vi "Step 8.vi"(8 "error in (no error)":errorcluster, 11 "HeatUp Data in":string[][](array[string])) -> (0 "error out":errorcluster, 1 "Min-Run Evap Temp (T3A)":dbl, 2 "EEV":u32, 3 "Evaporator Superheat (Deg F)":dbl format="%#.4g", 4 "Evaporator Superheat":T1(graph), 5 "Min-Run Evap Temp (T3A)":T1(graph), 7 "EEV":T1(graph))   [LabVIEW 2019]
uses:
  <vilib>/Utility/error.llb/DialogType.ctl
panel:
  out "error out 2":errorcluster
  in  "error in (no error) 2":errorcluster
  out "120 Array":dbl[][](array[numeric])
  out "transposed array":dbl[][](array[numeric])
  out "HeatUp Data in 2":string[][](array[string])
  # "Data with Stripped Header"
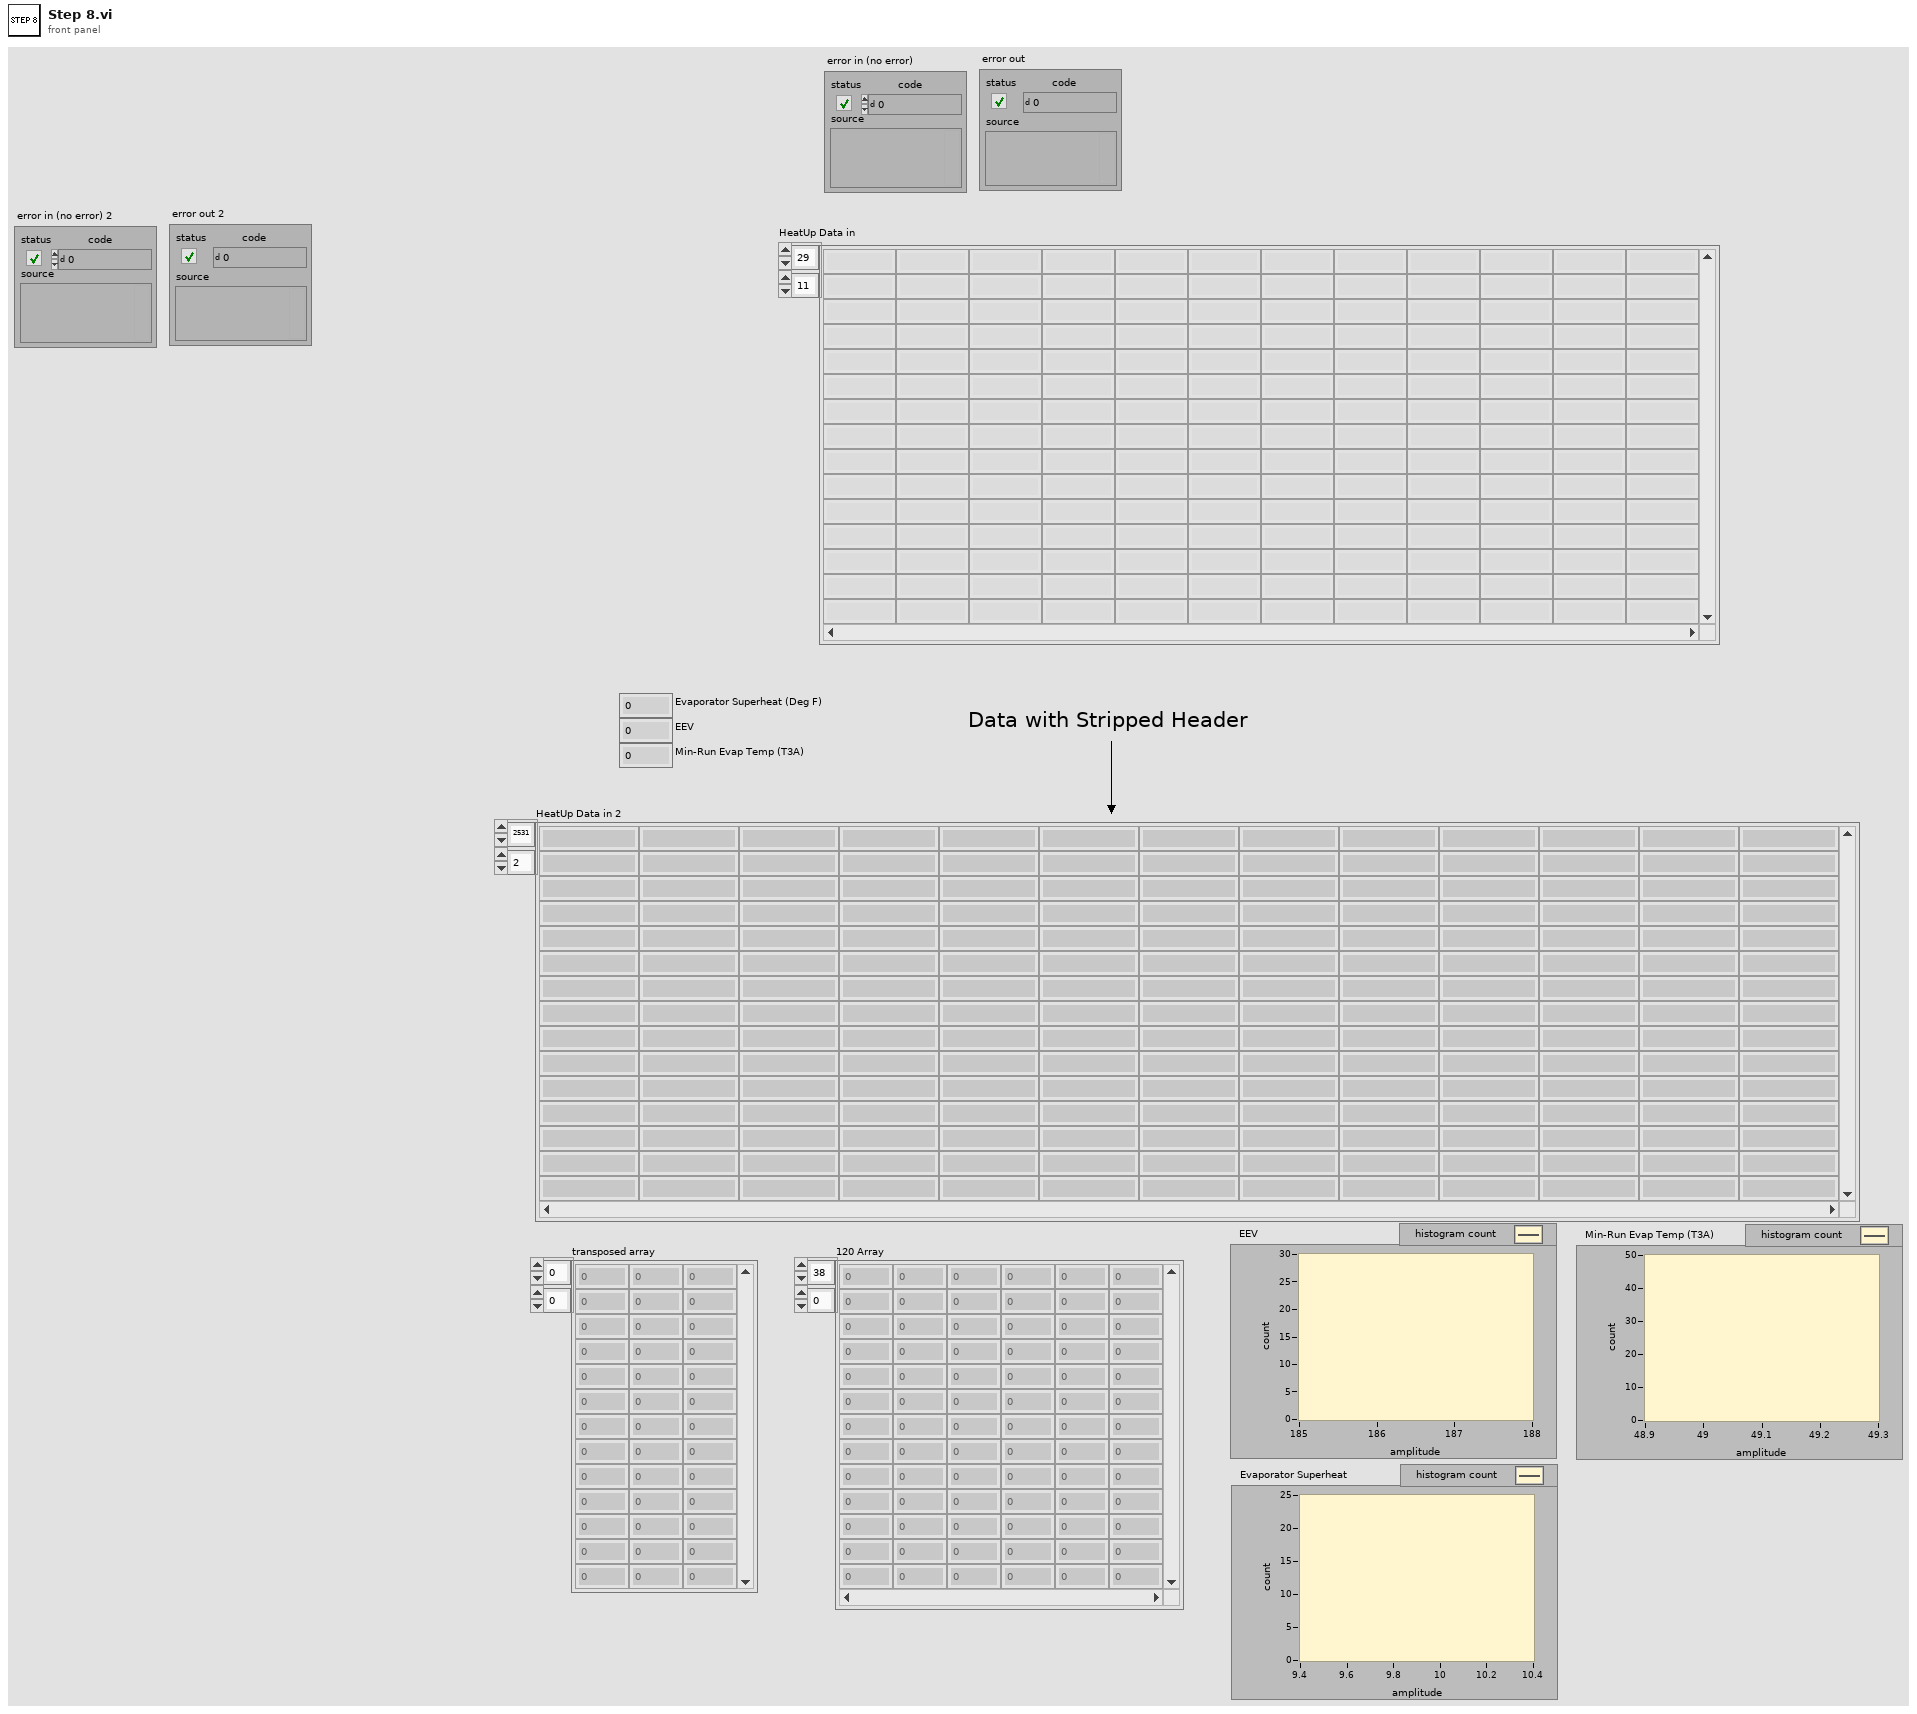
[diagram p1: front panel]
types:
  T1 = cluster{"X Values":dbl[], "Histogram: h(x)":i32[]}
  T2 = typedef "DialogType.ctl" = u16
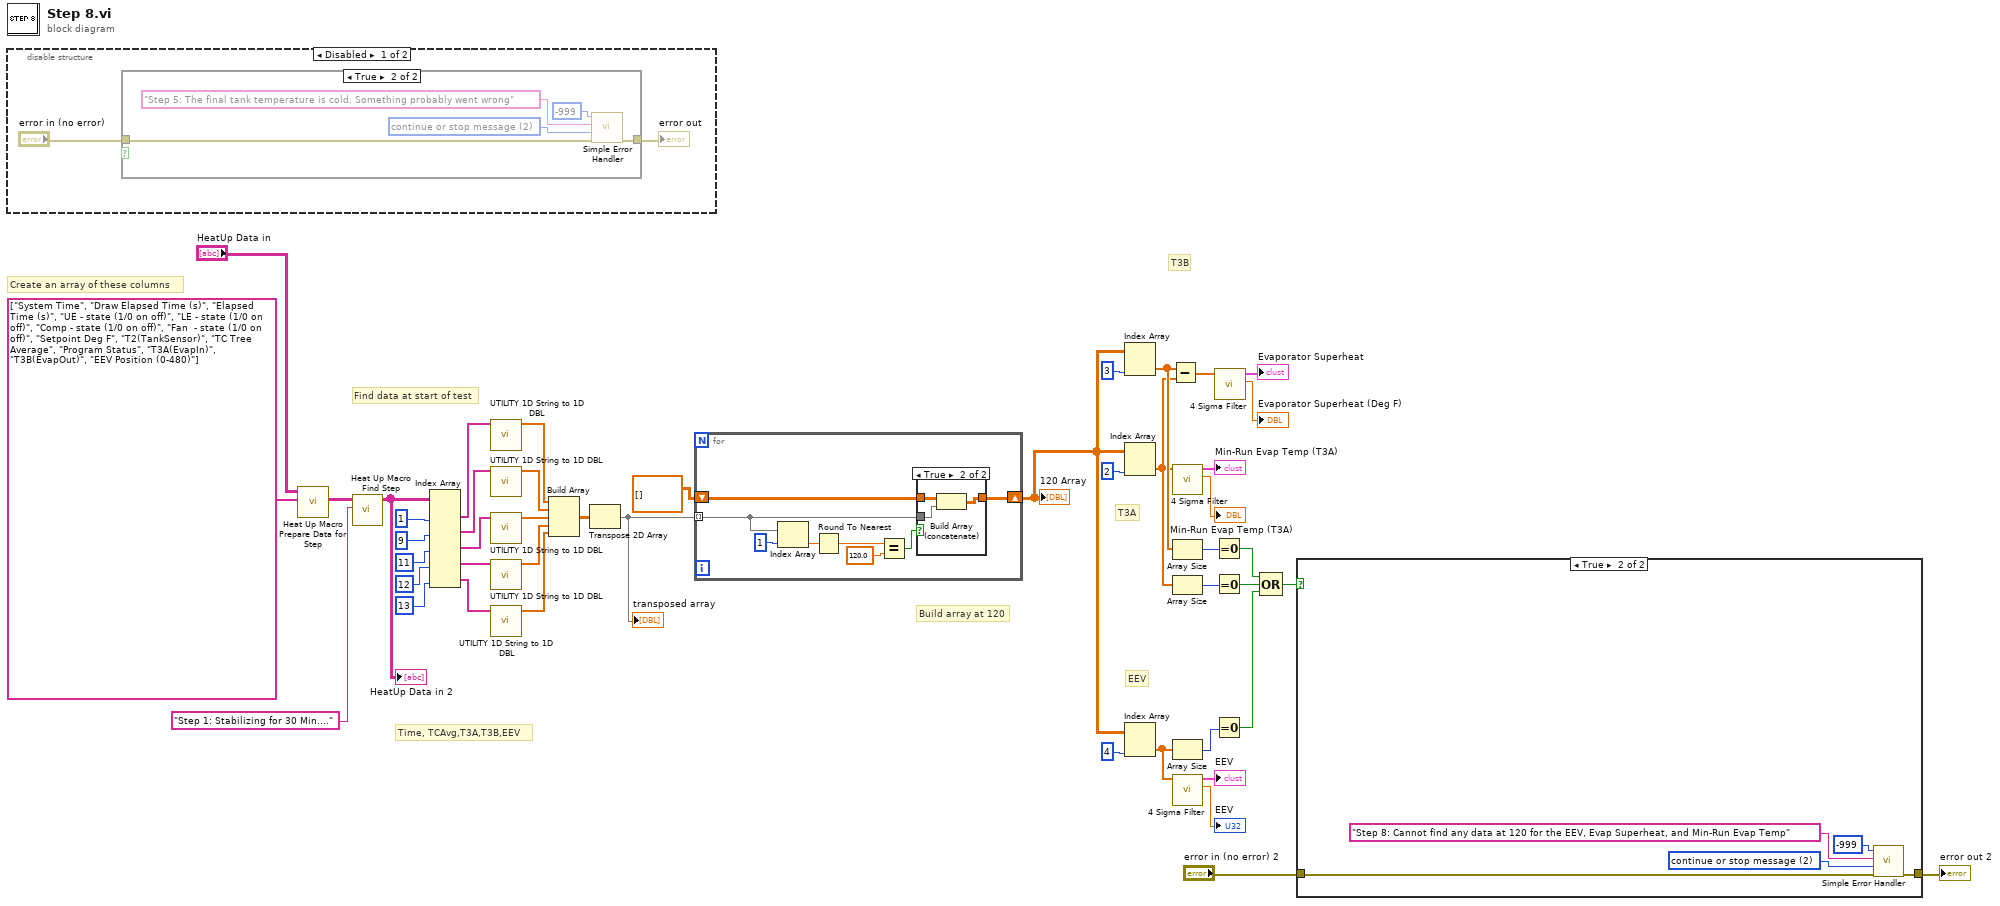
[diagram p0: block diagram]
diagram:
  # "Find data at start of test"
  # "EEV"
  # "Build array at 120"
  # "T3B"
  # "T3A"
  # "Time, TCAvg,T3A,T3B,EEV"
  # "Create an array of these columns"
  n1 = disable-structure shown="Disabled" {
    frame Disabled {
      n2 = case shown="True" {
        selector: _ -> [_ _]
        tunnel: "error in (no error)" -> [w49 w54]
        tunnel: [w49 w53] -> w47
        frame False {
        }
        frame True {
          w52 = T2 2 items=["no dialog", "OK message", "continue or stop message", "OK message + warnings", "continue/stop + warnings"] ("type of dialog (OK msg:1)")
          n3 = call <vilib>:"Simple Error Handler.vi"("error code (no error:0)"=-999, "error source (\" \")"="Step 5: The final tank temperature is cold. Something probably went wrong" ("error source (\" \")"), "type of dialog (OK msg:1)"=w52, "error in (no error)"=w54) -> ("error out"=w53:errorcluster)  [unwired: 1 in, 4 out]
        }
      }
      "error out" <- w47
    }
    frame Enabled {
    }
  }
  n4 = call "Heat Up Macro Prepare Data for Step.vi"("Columns Too Search For"=string[] ["System Time", "Draw Elapsed Time (s)", "Elapsed Time (s)", "UE - state (1/0 on off)", "LE - state (1/0 on off)", "Comp - state (1/0 on off)", "Fan  - state (1/0 on off)", "Setpoint Deg F", "T2(TankSensor)", "TC Tree Average", "Program Status", "T3A(EvapIn)", "T3B(EvapOut)", "EEV Position (0-480)"], "HeatUp Raw Data Input"="HeatUp Data in") -> ("Heat Up Data with Only Selected Columns"=w3:string[][])  [unwired: 8 in, 1 out]
  n5 = call "Heat Up Macro Find Step.vi"("Search For Step Name"="Step 1: Stabilizing for 30 Min...." ("y"), "Heat Up Data with Only Selected Columns"=w3) -> ("Filtered Array"=w1:string[][])  [unwired: 7 in, 2 out]
  "HeatUp Data in 2" <- w1
  n6 = Index Array(array=w1, index (col) #1=1 ("disabled index (col)"), index (col) #2=9 ("index (col)"), index (col) #3=11 ("index (col)"), index (col) #4=12 ("index (col)"), index (col) #5=13 ("index (col)")) -> (element #1=w43:string[], element #2=w42:string[], element #3=w41:string[], element #4=w30:string[], element #5=w29:string[])  [unwired: 5 in]
  n7 = call "UTILITY 1D String to 1D DBL.vi"("Save Data"=w43) -> ("DBL"=w40:dbl[])  [unwired: 10 in]
  n8 = call "UTILITY 1D String to 1D DBL.vi"("Save Data"=w42) -> ("DBL"=w39:dbl[])  [unwired: 10 in]
  n9 = call "UTILITY 1D String to 1D DBL.vi"("Save Data"=w41) -> ("DBL"=w38:dbl[])  [unwired: 10 in]
  n10 = call "UTILITY 1D String to 1D DBL.vi"("Save Data"=w30) -> ("DBL"=w28:dbl[])  [unwired: 10 in]
  n11 = call "UTILITY 1D String to 1D DBL.vi"("Save Data"=w29) -> ("DBL"=w27:dbl[])  [unwired: 10 in]
  n12 = Build Array(w40, w39, w38, w28, w27) -> (w37:dbl[][])
  n13 = Transpose 2D Array(2D array=w37) -> (transposed array=w36:dbl[][])
  "transposed array" <- w36
  n14 = for {
    tunnel: w36 -> [w58] mode=indexing
    shift-right: [w60] -> w26
    shift-left: dbl[][] [] -> [w61]
    n15 = Index Array(array=w58, index=1) -> (element=w59:dbl)
    n16 = Round To Nearest(number=w59) -> (nearest integer value=w56:dbl)
    n17 = Equal?(x=w56, y=120.0) -> (x = y?=w55:bool)
    n18 = case shown="True" w55 {
      tunnel: w61 -> [w63 w66]
      tunnel: [w63 w65] -> w60
      tunnel: w58 -> [_ w64]
      frame False {
      }
      frame True {
        n19 = Build Array (concatenate)(w66, w64) -> (w65:dbl[][])
      }
    }
  }
  "120 Array" <- w26
  n20 = Index Array(array=w26, index (col)=3 ("disabled index (col)")) -> (element=w15:dbl[])  [unwired: 1 in]
  n21 = Index Array(array=w26, index (col)=2 ("disabled index (col)")) -> (element=w14:dbl[])  [unwired: 1 in]
  n22 = Index Array(array=w26, index (col)=4 ("disabled index (col)")) -> (element=w13:dbl[])  [unwired: 1 in]
  n23 = Subtract(x=w15, y=w14) -> (x-y=w21:dbl[])
  n24 = call "4 Sigma Filter.vi"("Input Data"=w14) -> ("mean"=→"Min-Run Evap Temp (T3A)":dbl, "Histogram Graph"=→"Min-Run Evap Temp (T3A)":T1)  [unwired: 9 in]
  n25 = Array Size(array=w15) -> (size(s)=w12:i32)
  n26 = Array Size(array=w14) -> (size(s)=w11:i32)
  n27 = Array Size(array=w13) -> (size(s)=w10:i32)
  n28 = call "4 Sigma Filter.vi"("Input Data"=w13) -> ("mean"=→"EEV":dbl, "Histogram Graph"=→"EEV":T1)  [unwired: 9 in]
  n29 = Equal To 0?(x=w12) -> (x = 0?=w9:bool)
  n30 = Equal To 0?(x=w11) -> (x = 0?=w8:bool)
  n31 = Equal To 0?(x=w10) -> (x = 0?=w7:bool)
  n32 = call "4 Sigma Filter.vi"("Input Data"=w21) -> ("mean"=→"Evaporator Superheat (Deg F)":dbl, "Histogram Graph"=→"Evaporator Superheat":T1)  [unwired: 9 in]
  n33 = Compound Arithmetic op=OR(w9, w8, w7) -> (w6:bool)
  n34 = case shown="True" w6 {
    tunnel: "error in (no error) 2" -> [w67 w72]
    tunnel: [w67 w71] -> w16
    frame False {
    }
    frame True {
      w70 = T2 2 items=["no dialog", "OK message", "continue or stop message", "OK message + warnings", "continue/stop + warnings"] ("type of dialog (OK msg:1)")
      n35 = call <vilib>:"Simple Error Handler.vi"("error code (no error:0)"=-999, "error source (\" \")"="Step 8: Cannot find any data at 120 for the EEV, Evap Superheat, and Min-Run Evap Temp" ("error source (\" \")"), "type of dialog (OK msg:1)"=w70, "error in (no error)"=w72) -> ("error out"=w71:errorcluster)  [unwired: 1 in, 4 out]
    }
  }
  "error out 2" <- w16
